vi "52-lfs-r5 begin.vi"(8 "error in (no error)":errorcluster, 9 "Position in":T1) -> (0 "error out":errorcluster, 1 "Position out":T1, 4 "side?":bool)   [LabVIEW 2019]
uses:
  subVI/move/position cluster.ctl
  subVI/move control/move and align/move_cluster.ctl
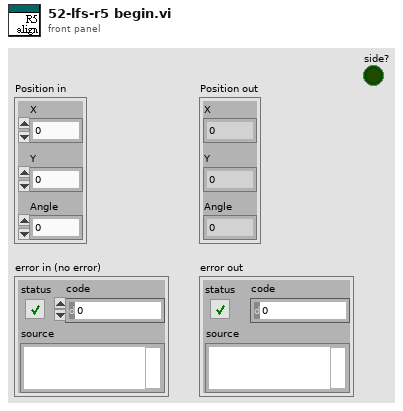
[diagram p1: front panel]
types:
  T1 = typedef "position cluster.ctl" = cluster{"X":dbl, "Y":dbl, "Angle":dbl}
  T2 = typedef "move_cluster.ctl" = cluster{"X":dbl, "Y":dbl, "degree":dbl, "speed":dbl}
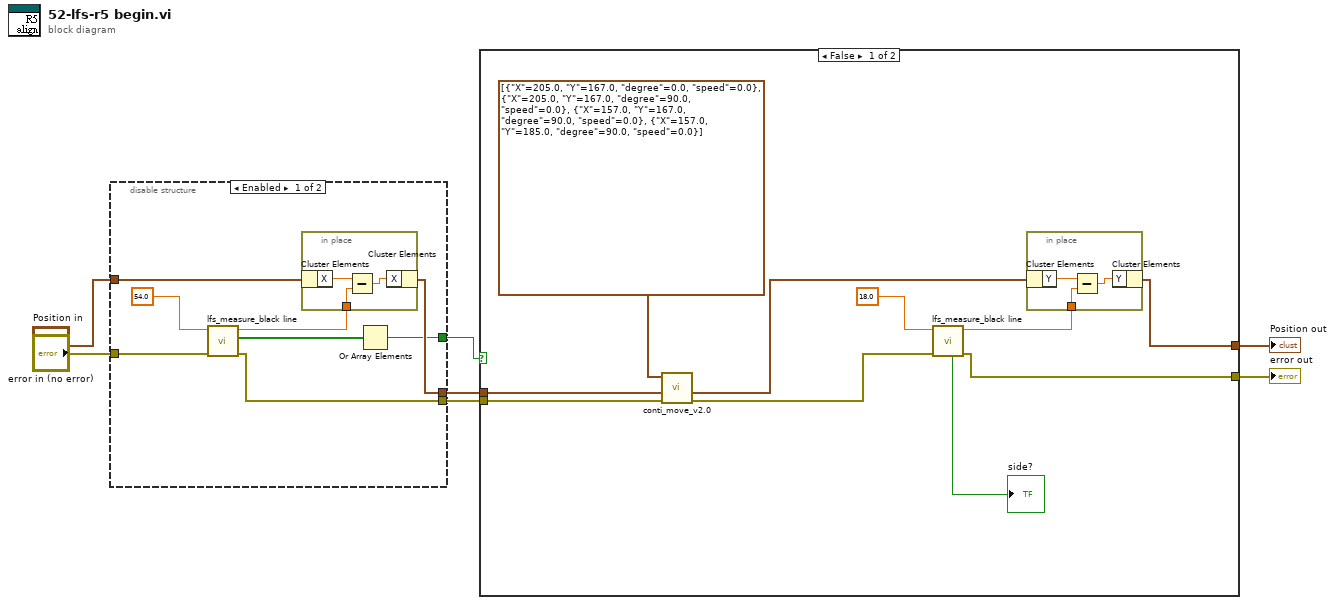
[diagram p0: block diagram]
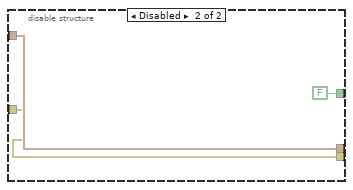
[diagram p2: hidden frame]
diagram:
  n1 = disable-structure shown="Enabled" {
    disable-tunnel: "error in (no error)" -> [w15 w20]
    disable-tunnel: "Position in" -> [w14 w21]
    disable-tunnel: [w10 w20] -> w5
    disable-tunnel: [w9 w21] -> w4
    disable-tunnel: [w8 FALSE] -> w1
    frame Enabled {
      n2 = call "lfs_measure_black line.vi"("error in (no error)"=w15, "limit"=54.0) -> ("error out"=w10:errorcluster, "0:R 1:L"=w11:bool[], "move cm"=w12:dbl)  [unwired: 6 in, 1 out]
      n3 = in-place {
        in-place-border: w12 -> [w18]
        n4 = in-place-cluster #1(w14) -> ("X"=w16:dbl)
        n5 = Subtract(x=w16, y=w18) -> (x-y=w17:dbl)
        n6 = in-place-cluster #1("X"=w17) -> (w9:T1)
      }
      n7 = Or Array Elements(Boolean array=w11) -> (logical OR=w8:bool)
    }
    frame Disabled {
    }
  }
  n8 = case shown="False" w1 {
    tunnel: w5 -> [w29 w35]
    tunnel: w4 -> [w24 w36]
    tunnel: [w28 w35] -> w3
    tunnel: [w27 w36] -> w2
    frame False {
      n9 = call "conti_move_v2.0.vi"("error in (no error)"=w29, "Position"=w24, "route"=T2[] [{"X"=205.0, "Y"=167.0, "degree"=0.0, "speed"=0.0}, {"X"=205.0, "Y"=167.0, "degree"=90.0, "speed"=0.0}, {"X"=157.0, "Y"=167.0, "degree"=90.0, "speed"=0.0}, {"X"=157.0, "Y"=185.0, "degree"=90.0, "speed"=0.0}]) -> ("error out"=w26:errorcluster, "Position out"=w25:T1)  [unwired: 7 in]
      n10 = call "lfs_measure_black line.vi"("error in (no error)"=w26, "limit"=18.0) -> ("error out"=w28:errorcluster, "move cm"=w31:dbl, "side?"=→"side?":bool)  [unwired: 6 in, 1 out]
      n11 = in-place {
        in-place-border: w31 -> [w34]
        n12 = in-place-cluster #2(w25) -> ("Y"=w32:dbl)
        n13 = Subtract(x=w32, y=w34) -> (x-y=w33:dbl)
        n14 = in-place-cluster #2("Y"=w33) -> (w27:T1)
      }
    }
    frame True {
    }
  }
  "Position out" <- w2
  "error out" <- w3
